vi "CRYCal points interp warning.vi"(9 "Device":u16, 10 "Sine waves":cluster{"freq":dbl, "ampl":dbl, "cycles":dbl}[](array[cluster]) {"cycles" format="%.2f"; "ampl" format="%.2f"; "freq" format="%.2f"}, 11 "Equalization":cluster{"Hz":dbl, dbl, "Deg":dbl}[](array[cluster])=[{"Hz"=1.0, 1.0, "Deg"=0.0}, {"Hz"=20000.0, 1.0, "Deg"=0.0}] {"Deg" format="%.1f"; "?" format="%.1f"}) -> ()   [LabVIEW 2013]
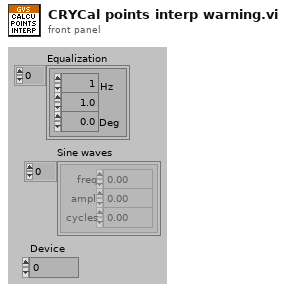
[diagram p1: front panel]
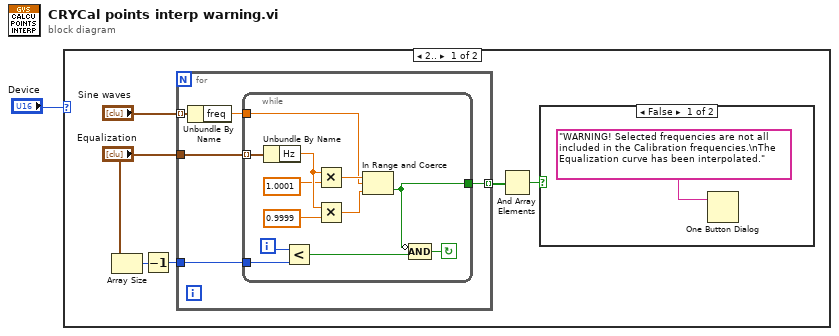
[diagram p0: block diagram]
diagram:
  n1 = case shown="2.." "Device" {
    frame 2.. {
      n2 = Array Size(array="Equalization") -> (size(s)=w5:i32)
      n3 = Decrement(x=w5) -> (x-1=w4:i32)
      n4 = for {
        tunnel: "Sine waves" -> [w13] mode=indexing
        tunnel: "Equalization" -> [w12]
        tunnel: w4 -> [w11]
        tunnel: [w9] -> w3 mode=indexing
        n5 = Unbundle By Name(w13) -> ("freq"=w10:dbl)
        n6 = while {
          tunnel: w12 -> [w25] mode=indexing
          tunnel: w11 -> [w18]
          tunnel: w10 -> [w19]
          tunnel: [w14] -> w9
          i -> [w17]
          stop <- w15 continue-if-true
          n7 = Unbundle By Name(w25) -> ("Hz"=w24:dbl)
          n8 = Less?(x=w17, y=w18) -> (x < y?=w16:bool)
          n9 = Multiply(x=w24, y=1.0001) -> (x*y=w21:dbl)
          n10 = Multiply(x=w24, y=0.9999) -> (x*y=w20:dbl)
          n11 = In Range and Coerce(upper limit=w21, x=w19, lower limit=w20) -> (In Range?=w14:bool)  [unwired: 1 out]
          n12 = Compound Arithmetic op=AND(invert w14, w16) -> (w15:bool)
        }
      }
      n13 = And Array Elements(Boolean array=w3) -> (logical AND=w2:bool)
      n14 = case shown="False" w2 {
        frame False {
          n15 = One Button Dialog(message="WARNING! Selected frequencies are not all included in the Calibration frequencies.\nThe Equalization curve has been interpolated.") -> ()  [unwired: 2 out]
        }
        frame True {
        }
      }
    }
    frame Default {
    }
  }
